vi "to_json.vi"(8 "error in":errorcluster, 11 "payload in":refnum<class "payload.lvclass">) -> (0 "error out":errorcluster, 2 "json":string, 3 "payload out":refnum<class "payload.lvclass">)   [LabVIEW 2020, in "datasources.lvlib" / "payload.lvclass"]
uses:
  payload.lvclass
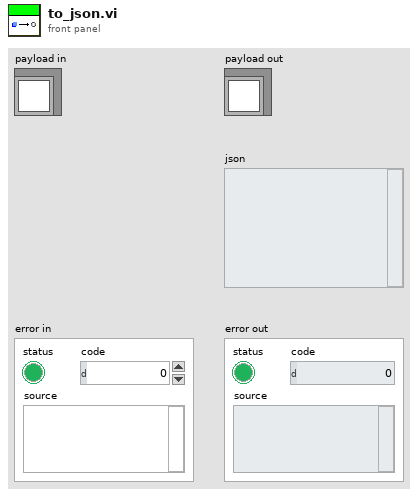
[diagram p1: front panel]
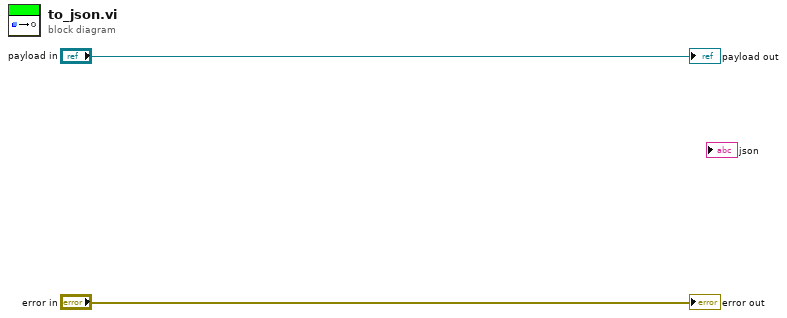
[diagram p0: block diagram]
diagram:
  "payload out" <- "payload in"
  "error out" <- "error in"
